vi "LDT Telescope Watch Dog.vi"(11 "XML String":string) -> (3 "Connected":bool)   [LabVIEW 2022 SP3, in "LDT Telescope.lvclass"]
uses:
  LDT Telescope.lvclass
  LDT Telescope.lvclass/LDT Telescope.ctl
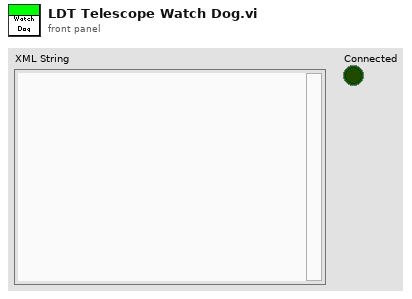
[diagram p1: front panel]
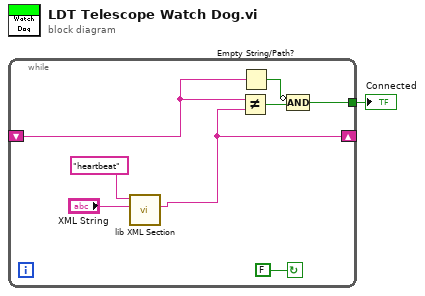
[diagram p0: block diagram]
diagram:
  n1 = while {
    shift-right: [w6] -> _
    shift-left: _ -> [w5]
    tunnel: [w2] -> w1
    stop <- FALSE continue-if-true
    n2 = call "lib XML Section.vi"("XML String"="XML String", "XML Topic"="heartbeat") -> ("XML Topic Body"=w6:string)  [unwired: 7 in, 2 out]
    n3 = Not Equal?(x=w5, y=w6) -> (x != y?=w4:bool)
    n4 = Empty String/Path?(string/path=w5) -> (empty?=w3:bool)
    n5 = Compound Arithmetic op=AND(invert w3, w4) -> (w2:bool)
  }
  "Connected" <- w1
